vi "Get Exported DPIDs.vi"(8 "error in (no error)":errorcluster, 10 "DPIDs GUID":string, 11 "Section Ref in":T1 format="%.0x") -> (0 "error out":errorcluster, 2 "DPIDs":T2, 3 "Section Ref out":T1 format="%.0x")   [LabVIEW 2013, in "Diagnostics Addon System Explorer.lvlib"]
uses:
  Diagnostics Addon System Explorer.lvlib
  <vilib>/NI Veristand/Custom Device API/Custom Device Item Ref.ctl
  Exported DPIDs Cluster.ctl
  Exported DPID Parameters.ctl
  Shared/DPID Parameters.ctl
  Shared/DPID Periodic Rate.ctl
  Shared/FG Action.ctl
  <vilib>/NI Veristand/Custom Device Tools/Custom Device Utility Library/NI VeriStand - Search for Item by GUID.vi
  Shared/GUID Lookup.vi
  <vilib>/NI Veristand/Custom Device API/NI VeriStand - Get Item Property.vi
  <vilib>/NI Veristand/Custom Device API/Get Item Property (Variant).vi
  <vilib>/NI Veristand/Custom Device Tools/Custom Device Utility Library/Custom Device Utility Library.lvlib
  Shared/Diagnostics Addon Shared.lvlib
  <vilib>/NI Veristand/Custom Device API/Custom Device API.lvlib
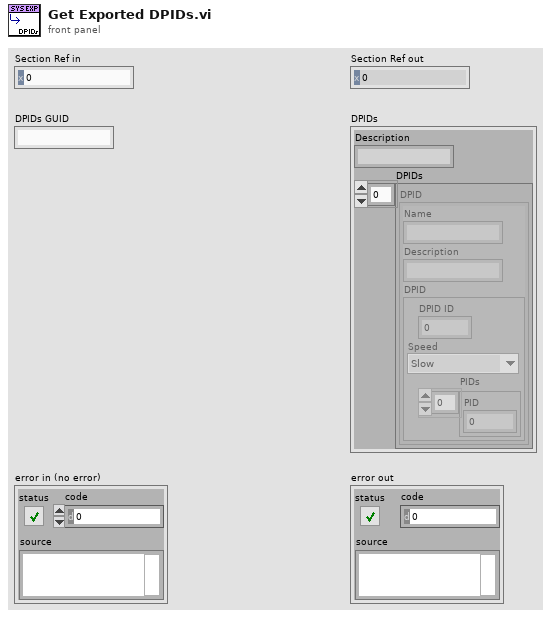
[diagram p1: front panel]
types:
  T1 = typedef "Custom Device API.lvlib/Custom Device Item Ref.ctl" = u64
  T2 = typedef "Diagnostics Addon System Explorer.lvlib/Exported DPIDs Cluster.ctl" = cluster{"Description":string, "DPIDs":T3[]}
  T3 = typedef "Diagnostics Addon System Explorer.lvlib/Exported DPID Parameters.ctl" = cluster{"Name":string, "Description":string, "DPID":T4}
  T4 = typedef "Diagnostics Addon Shared.lvlib/DPID Parameters.ctl" = cluster{"DPID ID":u8, "Speed":T5, "PIDs":u16[]}
  T5 = typedef "Diagnostics Addon Shared.lvlib/DPID Periodic Rate.ctl" = enum16{"Slow", "Medium", "Fast"}
  T6 = typedef "Diagnostics Addon Shared.lvlib/FG Action.ctl" = enum16{"Get", "Set"}
  T7 = typedef "Custom Device API.lvlib/Custom Device Item Info.ctl" = cluster{"Name":string, "Is Channel":bool, "GUID":string, "Is Waveform":bool}
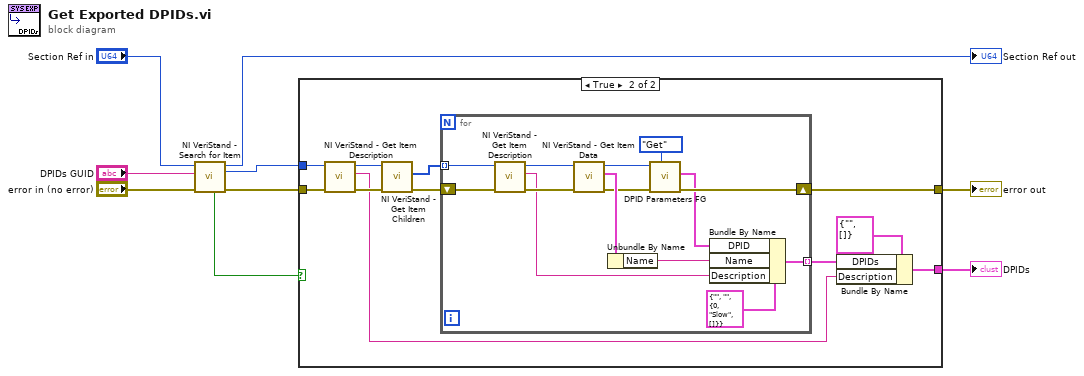
[diagram p0: block diagram]
diagram:
  n1 = call-poly <vilib>:"NI VeriStand - Search for Item.vi"("error in"="error in (no error)", "Item GUID"="DPIDs GUID", "Section Ref in"="Section Ref in") -> ("error out"=w9:errorcluster, "Item Ref"=w8:T1, "Section Ref out"=→"Section Ref out":T1, "Found"=w7:bool)  [unwired: 5 in]
  n2 = case shown="True" w7 {
    tunnel: w8 -> [_ w16]
    tunnel: w9 -> [w10 w17]
    tunnel: [w10 w20] -> w5
    tunnel: [_ w11] -> w4
    frame False {
    }
    frame True {
      n3 = call <vilib>:"NI VeriStand - Get Item Description.vi"("error in (no error)"=w17, "Item Ref in"=w16) -> ("error out"=w14:errorcluster, "Description"=w13:string, "Item Ref out"=w15:T1)  [unwired: 7 out]
      n4 = call <vilib>:"NI VeriStand - Get Item Children.vi"("error in (no error)"=w14, "Item Ref in"=w15) -> ("error out"=w21:errorcluster, "Child Refs"=w19:T1[])  [unwired: 6 in, 2 out]
      n5 = for {
        tunnel: w19 -> [w31] mode=indexing
        tunnel: [w28] -> w12 mode=indexing
        shift-right: [w25] -> w20
        shift-left: w21 -> [w32]
        n6 = call <vilib>:"NI VeriStand - Get Item Description.vi"("error in (no error)"=w32, "Item Ref in"=w31) -> ("error out"=w34:errorcluster, "Description"=w29:string, "Item Ref out"=w33:T1)  [unwired: 7 out]
        n7 = call <vilib>:"NI VeriStand - Get Item Data.vi"("error in (no error)"=w34, "Item Ref in"=w33) -> ("error out"=w27:errorcluster, "Item Info"=w35:T7, "Item Ref out"=w26:T1)  [unwired: 7 out]
        n8 = Unbundle By Name(w35) -> ("Name"=w30:string)
        n9 = call "DPID Parameters FG.vi"("Action"=FG_Action."Get", "error in (no error)"=w27, "Device Item Ref in"=w26) -> ("error out"=w25:errorcluster, "DPID"=w22:T4)  [unwired: 6 in, 1 out]
        n10 = Bundle By Name(cluster=T3 {"Name"="", "Description"="", "DPID"={"DPID ID"=0, "Speed"=enum."Slow", "PIDs"=[]}} ("DPID"), "DPID"=w22, "Name"=w30, "Description"=w29) -> (w28:T3)
      }
      n11 = Bundle By Name(cluster=T2 {"Description"="", "DPIDs"=[]}, "DPIDs"=w12, "Description"=w13) -> (w11:T2)
    }
  }
  "error out" <- w5
  "DPIDs" <- w4
